vi "Measurement.Free.ReftoDVR.vi"(10 "Ref":u32 format="%08x") -> (2 "Ref":T1)   [LabVIEW 2017, in "Measurement.Free.lvclass"]
doc: "JKI State Machine Objects (SMO) 1.0.0.5\nJKI - JKI\nCopyright (c) 2016, JKI"
uses:
  Measurement.Free.lvclass
  Typedefs/Configuration--Cluster.ctl
  Typedefs/PrivateData--Cluster.ctl
  Typedefs/PrivateData--Ref.ctl
  OPA/Typedefs/Configuration--Cluster.ctl
  OPA/OPA.lvclass
  Measurement/Typedefs/Configuration.OPA--Cluster.ctl
  Measurement/Measurement.lvclass
  OPM/Typedefs/Configuration--Cluster.ctl
  OPM/OPM.lvclass
  Measurement/Typedefs/Configuration.OPM--Cluster.ctl
  LIA/Typedefs/Configuration--Cluster.ctl
  LIA/LIA.lvclass
  Measurement/Typedefs/Configuration.LIA--Cluster.ctl
  SMU/Typedefs/Configuration--Cluster.ctl
  SMU/SMU.lvclass
  Measurement/Typedefs/Configuration.SMU--Cluster.ctl
  Typedefs/Configuration.Hardware--Cluster.ctl
  Typedefs/Dependencies--Cluster.ctl
  Typedefs/PrivateEvents--Cluster.ctl
  Typedefs/PrivateEvents--Measurement.Free.SMU.SetVoltage.ctl
  Typedefs/PrivateEvents--Measurement.Free.OPA.SetWavelength.ctl
  Typedefs/PrivateEvents--Measurement.Free.OPA.SetShutterState.ctl
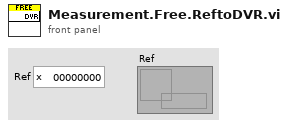
[diagram p1: front panel]
types:
  T1 = typedef "Measurement.Free.lvclass/PrivateData--Ref.ctl" = refnum<data-value>
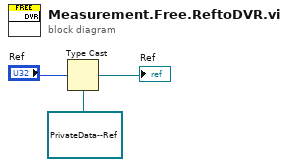
[diagram p0: block diagram]
diagram:
  n1 = Type Cast(type=T1 refnum ("Ref"), x="Ref") -> (*(type *) &x=→"Ref":T1)
